vi "AutoIndexing.vi"() -> ()   [LabVIEW 2011]
panel:
  out "Y":dbl[](array[numeric])
  in  "X":dbl[](array[numeric])=[1.0, 2.0, 3.0, 4.0]
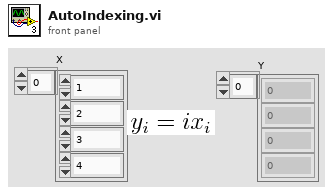
[diagram p1: front panel]
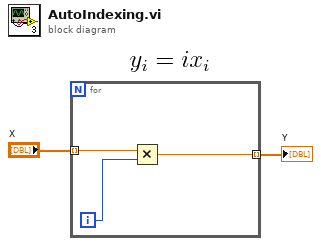
[diagram p0: block diagram]
diagram:
  n1 = for {
    tunnel: "X" -> [w5] mode=indexing
    tunnel: [w3] -> w1 mode=indexing
    i -> [w4]
    n2 = Multiply(x=w5, y=w4) -> (x*y=w3:dbl)
  }
  "Y" <- w1
